vi "S2C_PCIe7841_Proc_PortRead.vi"(8 "Error In":errorcluster, 11 "Data":string) -> (0 "Error Out":errorcluster, 3 "Port":string)   [LabVIEW 2015]
uses:
  Typedefs/S2C_PCIe7841_Type_Connector.ctl
  Typedefs/S2C_PCIe7841_Type_Port.ctl
  S2C_PCIe7841_Proc_Globals.vi
  <vilib>/Utility/error.llb/Error Cluster From Error Code.vi
  <vilib>/rvi/errors/niLvFpgaAdjustHostInterfaceError.vi
  <vilib>/rvi/interface/nirviReadWriteControl/nirviReadWriteControl.xnode
  NiFpgaLv.dll
  <vilib>/rvi/interface/Simulation/niFpgaSimulationCallBeginRW.vi
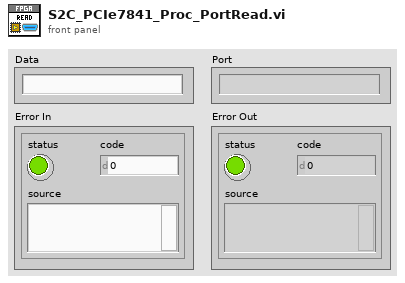
[diagram p1: front panel]
types:
  T1 = typedef "S2C_PCIe7841_Type_Connector.ctl" = u16
  T2 = typedef "S2C_PCIe7841_Type_Port.ctl" = u16
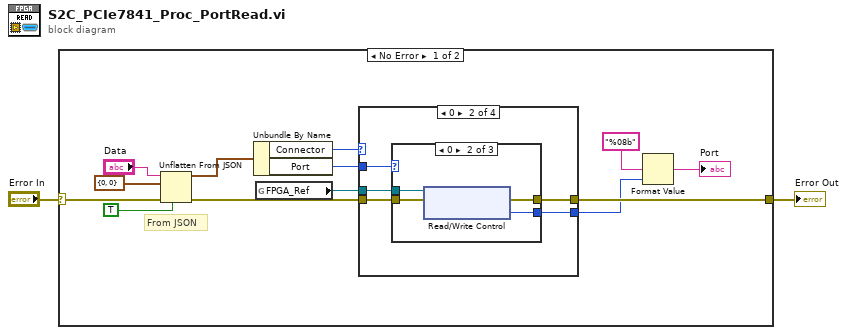
[diagram p0: block diagram]
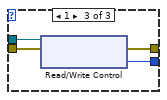
[diagram p4: hidden frame]
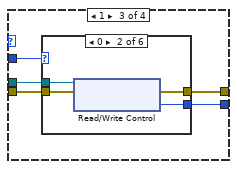
[diagram p5: hidden frame]
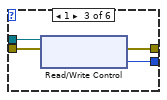
[diagram p7: hidden frame]
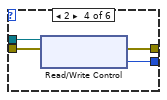
[diagram p8: hidden frame]
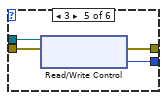
[diagram p9: hidden frame]
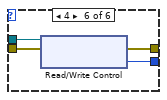
[diagram p10: hidden frame]
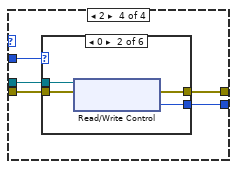
[diagram p11: hidden frame]
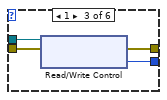
[diagram p13: hidden frame]
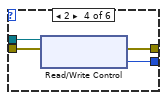
[diagram p14: hidden frame]
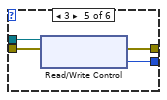
[diagram p15: hidden frame]
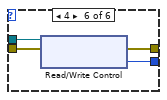
[diagram p16: hidden frame]
diagram:
  n1 = case shown="No Error" "Error In" {
    selector: "Error In" -> [w15 w83]
    tunnel: [w6 w83] -> w1
    frame No Error {
      # "From JSON"
      n2 = Unflatten From JSON(JSON string="Data", type and defaults=cluster{"Connector":T1, "Port":T2} {"Connector"=0, "Port"=0}, default null elements? (F)=TRUE, error in (no error)=w15) -> (value=w13:cluster{"Connector":T1, "Port":T2}, error out=w8:errorcluster)  [unwired: 3 in]
      n3 = Unbundle By Name(w13) -> ("Connector"=w10:T1, "Port"=w9:T2)
      n4 = global read "S2C_PCIe7841_Proc_Globals.vi" "FPGA_Ref"() -> (w7:refnum<k20>)
      n5 = case shown="0" w10 {
        tunnel: w9 -> [_ w19 w33 w59]
        tunnel: w8 -> [w16 w21 w35 w61]
        tunnel: w7 -> [_ w20 w34 w60]
        tunnel: [_ w18 w32 w58] -> w4
        tunnel: [w16 w17 w31 w57] -> w6
        frame 5, Default {
        }
        frame 0 {
          n6 = case shown="0" w19 {
            tunnel: w21 -> [w22 w26 w30]
            tunnel: w20 -> [_ w25 w29]
            tunnel: [_ w24 w28] -> w18
            tunnel: [w22 w23 w27] -> w17
            frame 5, Default {
            }
            frame 0 {
              n7 = xnode "Read/Write Control"("FPGA VI Reference In"=w25, "error in"=w26) -> ("error out"=w23:errorcluster, "Conn0/Port0"=w24:u8)  [unwired: 1 out]
            }
            frame 1 {
              n8 = xnode "Read/Write Control"("FPGA VI Reference In"=w29, "error in"=w30) -> ("error out"=w27:errorcluster, "Conn0/Port1"=w28:u8)  [unwired: 1 out]
            }
          }
        }
        frame 1 {
          n9 = case shown="0" w33 {
            tunnel: w35 -> [w36 w40 w44 w48 w52 w56]
            tunnel: w34 -> [_ w39 w43 w47 w51 w55]
            tunnel: [_ w38 w42 w46 w50 w54] -> w32
            tunnel: [w36 w37 w41 w45 w49 w53] -> w31
            frame 5, Default {
            }
            frame 0 {
              n10 = xnode "Read/Write Control"("FPGA VI Reference In"=w39, "error in"=w40) -> ("error out"=w37:errorcluster, "Conn1/Port0"=w38:u8)  [unwired: 1 out]
            }
            frame 1 {
              n11 = xnode "Read/Write Control"("FPGA VI Reference In"=w43, "error in"=w44) -> ("error out"=w41:errorcluster, "Conn1/Port1"=w42:u8)  [unwired: 1 out]
            }
            frame 2 {
              n12 = xnode "Read/Write Control"("FPGA VI Reference In"=w47, "error in"=w48) -> ("error out"=w45:errorcluster, "Conn1/Port2"=w46:u8)  [unwired: 1 out]
            }
            frame 3 {
              n13 = xnode "Read/Write Control"("FPGA VI Reference In"=w51, "error in"=w52) -> ("error out"=w49:errorcluster, "Conn1/Port3"=w50:u8)  [unwired: 1 out]
            }
            frame 4 {
              n14 = xnode "Read/Write Control"("FPGA VI Reference In"=w55, "error in"=w56) -> ("error out"=w53:errorcluster, "Conn1/Port4"=w54:u8)  [unwired: 1 out]
            }
          }
        }
        frame 2 {
          n15 = case shown="0" w59 {
            tunnel: w61 -> [w62 w66 w70 w74 w78 w82]
            tunnel: w60 -> [_ w65 w69 w73 w77 w81]
            tunnel: [_ w64 w68 w72 w76 w80] -> w58
            tunnel: [w62 w63 w67 w71 w75 w79] -> w57
            frame 5, Default {
            }
            frame 0 {
              n16 = xnode "Read/Write Control"("FPGA VI Reference In"=w65, "error in"=w66) -> ("error out"=w63:errorcluster, "Conn2/Port0"=w64:u8)  [unwired: 1 out]
            }
            frame 1 {
              n17 = xnode "Read/Write Control"("FPGA VI Reference In"=w69, "error in"=w70) -> ("error out"=w67:errorcluster, "Conn2/Port1"=w68:u8)  [unwired: 1 out]
            }
            frame 2 {
              n18 = xnode "Read/Write Control"("FPGA VI Reference In"=w73, "error in"=w74) -> ("error out"=w71:errorcluster, "Conn2/Port2"=w72:u8)  [unwired: 1 out]
            }
            frame 3 {
              n19 = xnode "Read/Write Control"("FPGA VI Reference In"=w77, "error in"=w78) -> ("error out"=w75:errorcluster, "Conn2/Port3"=w76:u8)  [unwired: 1 out]
            }
            frame 4 {
              n20 = xnode "Read/Write Control"("FPGA VI Reference In"=w81, "error in"=w82) -> ("error out"=w79:errorcluster, "Conn2/Port4"=w80:u8)  [unwired: 1 out]
            }
          }
        }
      }
      n21 = Format Value(format string="%08b", value (0)=w4) -> (output string=→"Port":string)  [unwired: 1 in]
    }
    frame Error {
    }
  }
  "Error Out" <- w1
